vi "find_config_files.vi"(11 "path":path) -> (3 "config files_names":string[](array[string]))   [LabVIEW 2013]
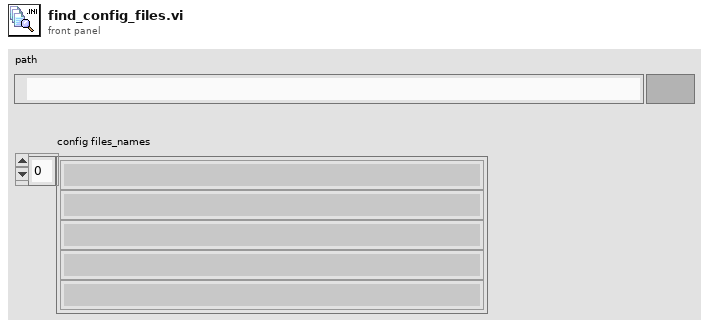
[diagram p1: front panel]
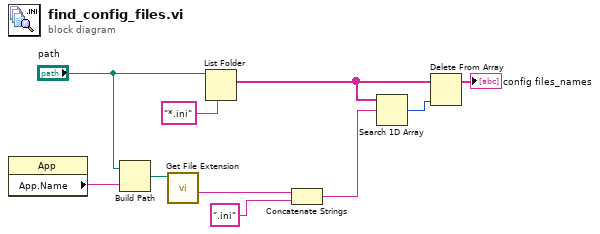
[diagram p0: block diagram]
diagram:
  n1 = property class="App"() -> ("App.Name"=w3:string)  [unwired: 2 in, 2 out]
  n2 = Build Path(base path="path", name or relative path=w3) -> (appended path=w2:path)
  n3 = call <vilib>:"Get File Extension.vi"("file"=w2) -> ("filename without extension"=w1:string)  [unwired: 7 in, 3 out]
  n4 = List Folder(path="path", pattern="*.ini") -> (filenames=w7:string[])  [unwired: 2 in, 3 out]
  n5 = Concatenate Strings(w1, ".ini" ("pattern")) -> (w6:string)
  n6 = Search 1D Array(1D array=w7, element=w6) -> (index of element=w8:i32)  [unwired: 1 in]
  n7 = Delete From Array(array=w7, index=w8) -> (array with subset deleted=→"config files_names":string[])  [unwired: 1 in, 1 out]
